vi "Build File Path.vi"(8 "error in (no error)":errorcluster, 10 "Time Stamp":timestamp, 11 "Log File Specification in":refnum<class "Log File Specification.lvclass">) -> (0 "error out":errorcluster, 2 "Instance File Path":path, 3 "Log File Specification out":refnum<class "Log File Specification.lvclass">)   [LabVIEW 2015, in "Log File Specification.lvclass"]
doc: "Builds an instance file path based on the specified path tag values and the <b>Time Stamp</b> parameter."
uses:
  Log File Specification.lvclass
  Log File Specification.lvclass/Log File Specification.ctl
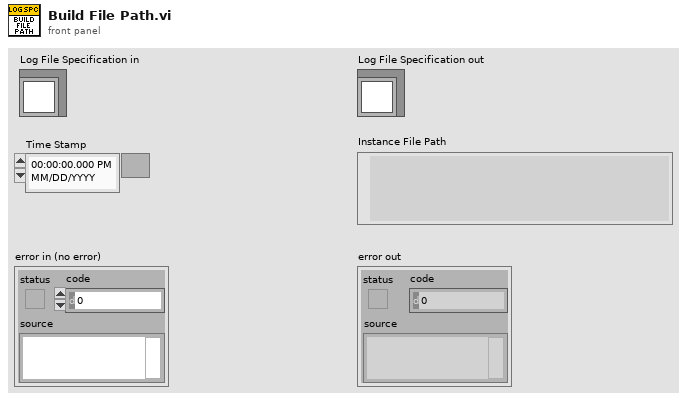
[diagram p1: front panel]
types:
  T1 = typedef "Log File Specification.lvclass/Path Segment.ctl" = cluster{"String":string, "Is Tag":bool}
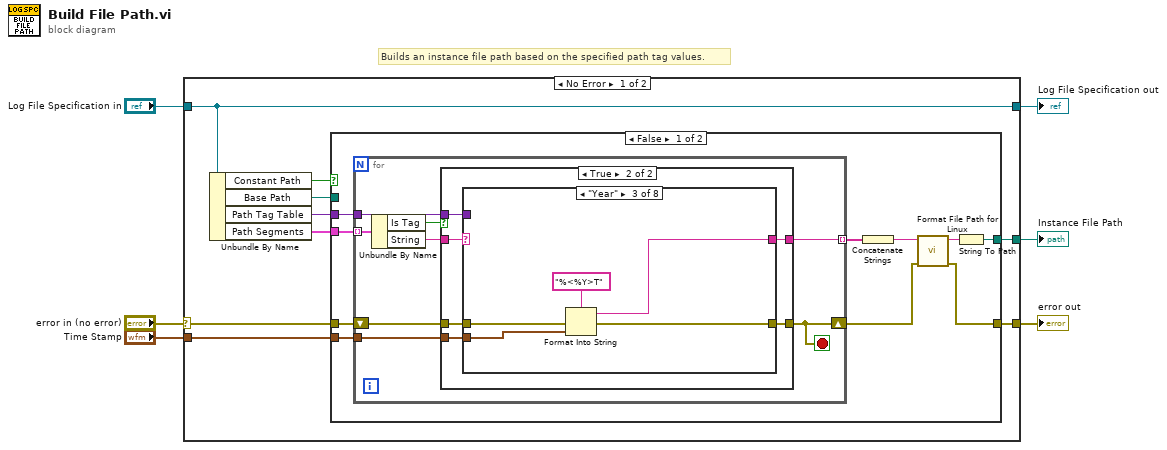
[diagram p0: block diagram]
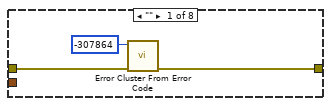
[diagram p3: hidden frame]
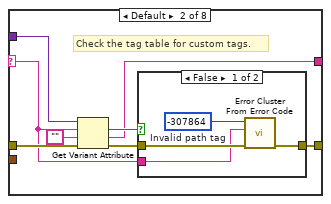
[diagram p4: hidden frame]
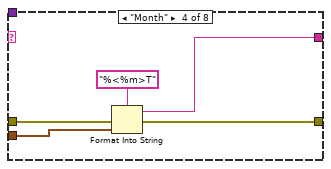
[diagram p6: hidden frame]
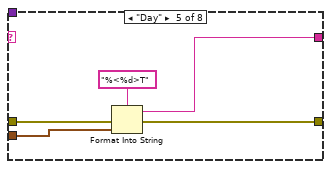
[diagram p7: hidden frame]
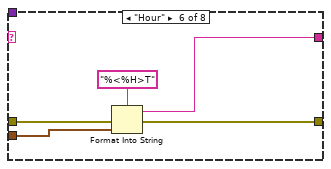
[diagram p8: hidden frame]
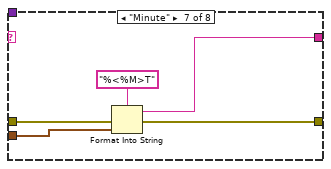
[diagram p9: hidden frame]
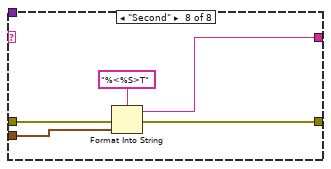
[diagram p10: hidden frame]
diagram:
  # "Builds an instance file path based on the specified path tag values."
  n1 = case shown="No Error" "error in (no error)" {
    selector: "error in (no error)" -> [w13 w91]
    tunnel: [w12 w91] -> w5
    tunnel: [w15 _] -> w1
    tunnel: "Time Stamp" -> [w11 _]
    tunnel: "Log File Specification in" -> [w9 w90]
    tunnel: [w9 w90] -> w2
    frame No Error {
      n2 = Unbundle By Name(w9) -> ("Constant Path"=w8:bool, "Base Path"=w7:path, "Path Tag Table"=w10:variant, "Path Segments"=w14:T1[])
      n3 = case shown="False" w8 {
        tunnel: [w25 w89] -> w15
        tunnel: w14 -> [w24 _]
        tunnel: w13 -> [w23 w88]
        tunnel: [w17 w88] -> w12
        tunnel: w11 -> [w22 _]
        tunnel: w10 -> [w20 _]
        tunnel: w7 -> [_ w89]
        frame False {
          n4 = for {
            tunnel: w24 -> [w33] mode=indexing
            shift-right: [w26] -> w18
            shift-left: w23 -> [w31]
            tunnel: w22 -> [w30]
            tunnel: [w29] -> w21 mode=indexing
            tunnel: w20 -> [w28]
            stop <- w26 stop-if-true
            n5 = Unbundle By Name(w33) -> ("Is Tag"=w32:bool, "String"=w27:string)
            n6 = case shown="True" w32 {
              tunnel: w27 -> [w34 w37]
              tunnel: w31 -> [w35 w40]
              tunnel: [w35 w39] -> w26
              tunnel: w28 -> [_ w38]
              tunnel: w30 -> [_ w36]
              tunnel: [w34 w41] -> w29
              frame False {
              }
              frame True {
                n7 = case shown="\"Year\"" w37 {
                  selector: w37 -> [_ w45 _ _ _ _ _ _]
                  tunnel: [_ w46 w59 w64 w69 w74 w79 w84] -> w41
                  tunnel: w40 -> [w44 w52 w62 w67 w72 w77 w82 w87]
                  tunnel: [w43 w48 w58 w63 w68 w73 w78 w83] -> w39
                  tunnel: w38 -> [_ w51 _ _ _ _ _ _]
                  tunnel: w36 -> [_ _ w61 w66 w71 w76 w81 w86]
                  frame "" {
                    n8 = call <vilib>:"Error Cluster From Error Code.vi"("error in (no error)"=w44, "error code (0)"=-307864) -> ("error out"=w43:errorcluster)  [unwired: 7 in]
                  }
                  frame Default {
                    # "Check the tag table for custom tags."
                    n9 = Get Variant Attribute(Variant=w51, name=w45, default value (empty Variant)="", error in=w52) -> (found=w49:bool, value=w46:string, error out=w47:errorcluster)  [unwired: 1 out]
                    n10 = case shown="False" w49 {
                      tunnel: [w54 w57] -> w48
                      tunnel: w47 -> [w55 w57]
                      tunnel: w45 -> [w53 _]
                      frame False {
                        w56 = -307864  # Invalid path tag
                        n11 = call <vilib>:"Error Cluster From Error Code.vi"("error in (no error)"=w55, "error message (\"\")"=w53, "error code (0)"=w56) -> ("error out"=w54:errorcluster)  [unwired: 6 in]
                      }
                      frame True {
                      }
                    }
                  }
                  frame "Year" {
                    n12 = Format Into String(format string="%<%Y>T", error in=w62, w61) -> (resulting string=w59:string, error out=w58:errorcluster)  [unwired: 1 in]
                  }
                  frame "Month" {
                    n13 = Format Into String(format string="%<%m>T", error in=w67, w66) -> (resulting string=w64:string, error out=w63:errorcluster)  [unwired: 1 in]
                  }
                  frame "Day" {
                    n14 = Format Into String(format string="%<%d>T", error in=w72, w71) -> (resulting string=w69:string, error out=w68:errorcluster)  [unwired: 1 in]
                  }
                  frame "Hour" {
                    n15 = Format Into String(format string="%<%H>T", error in=w77, w76) -> (resulting string=w74:string, error out=w73:errorcluster)  [unwired: 1 in]
                  }
                  frame "Minute" {
                    n16 = Format Into String(format string="%<%M>T", error in=w82, w81) -> (resulting string=w79:string, error out=w78:errorcluster)  [unwired: 1 in]
                  }
                  frame "Second" {
                    n17 = Format Into String(format string="%<%S>T", error in=w87, w86) -> (resulting string=w84:string, error out=w83:errorcluster)  [unwired: 1 in]
                  }
                }
              }
            }
          }
          n18 = Concatenate Strings(w21) -> (w19:string)
          n19 = call "Format File Path for Linux.vi"("error in (no error)"=w18, "Path"=w19) -> ("error out"=w17:errorcluster, "Path out"=w16:string)  [unwired: 8 in]
          n20 = String To Path(string=w16) -> (path=w25:path)
        }
        frame True {
          # "No tags to evaluate in the path."
        }
      }
    }
    frame Error {
    }
  }
  "Instance File Path" <- w1
  "error out" <- w5
  "Log File Specification out" <- w2
